vi "Wait For OPC.vi"(8 "error in":errorcluster, 10 "Timeout (10000 ms)":i32=10000, 11 "VISA resource name":refnum<visa-resource-name>) -> (0 "error out":errorcluster, 3 "VISA resource name out":refnum<visa-resource-name>)   [LabVIEW 2013, in "DmmPwr Simulator.lvlib"]
doc: "Waits for operation complete."
uses:
  <instrlib>/DmmPwr Simulator/DmmPwr Simulator.lvlib
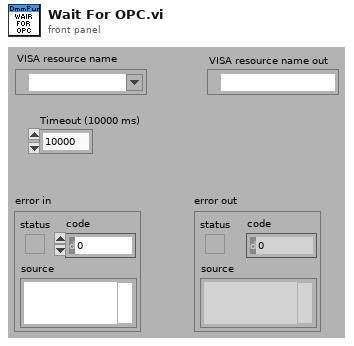
[diagram p1: front panel]
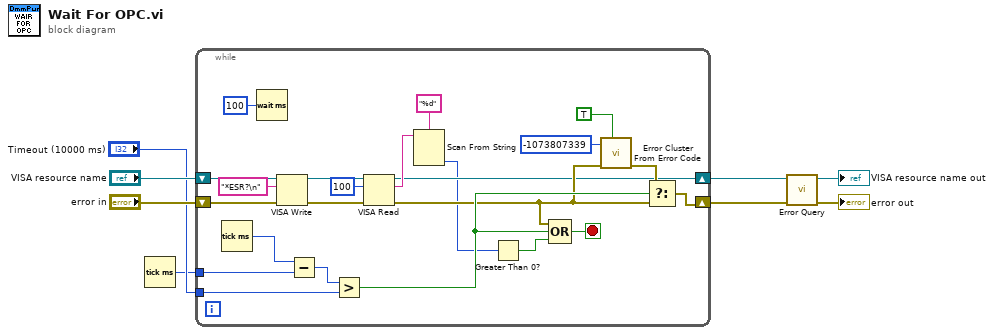
[diagram p0: block diagram]
diagram:
  n1 = Tick Count (ms)() -> (millisecond timer value=w1:u32)
  n2 = while {
    tunnel: "Timeout (10000 ms)" -> [w21]
    shift-right: [w17] -> w6
    shift-left: "error in" -> [w31]
    shift-right: [w13] -> w4
    shift-left: "VISA resource name" -> [w29]
    tunnel: w1 -> [w11]
    stop <- w19 stop-if-true
    n3 = Tick Count (ms)() -> (millisecond timer value=w23:u32)
    n4 = Wait (ms)(milliseconds to wait=u32 100) -> ()  [unwired: 1 out]
    n5 = VISA Write(VISA resource name=w29, write buffer="*ESR?\n", error in (no error)=w31) -> (VISA resource name out=w27:refnum<visa-resource-name>, error out=w28:errorcluster)  [unwired: 1 out]
    n6 = Subtract(x=w23, y=w11) -> (x-y=w22:u32)
    n7 = Greater?(x=w22, y=w21) -> (0:w18:bool)
    n8 = VISA Read(VISA resource name=w27, byte count=u32 100, error in (no error)=w28) -> (VISA resource name out=w13:refnum<visa-resource-name>, read buffer=w25:string, error out=w14:errorcluster)  [unwired: 1 out]
    n9 = Scan From String(format string="%d", input string=w25) -> (output 1=w9:i32)  [unwired: 3 in, 3 out]
    n10 = Greater Than 0?(x=w9) -> (x > 0?=w20:bool)
    n11 = Compound Arithmetic op=OR(w14, w18, w20) -> (w19:bool)
    n12 = call <vilib>:"Error Cluster From Error Code.vi"("show call chain? (False)"=TRUE, "error in (no error)"=w14, "error code (0)"=-1073807339) -> ("error out"=w16:errorcluster)  [unwired: 6 in]
    n13 = Select(t=w16, s=w18, f=w14) -> (s? t:f=w17:errorcluster)
  }
  n14 = call <instrlib>:"Error Query.vi"("error in (no error)"=w6, "VISA resource name"=w4) -> ("error out"=→"error out":errorcluster, "VISA resource name out"=→"VISA resource name out":refnum<visa-resource-name>)  [unwired: 6 in, 2 out]
